vi "ILABW_CaseHandler.vi"(2 "error In":errorcluster, 4 "data":string, 5 "action":string) -> (0 "errorOut":string, 1 "response":string)   [LabVIEW 2012]
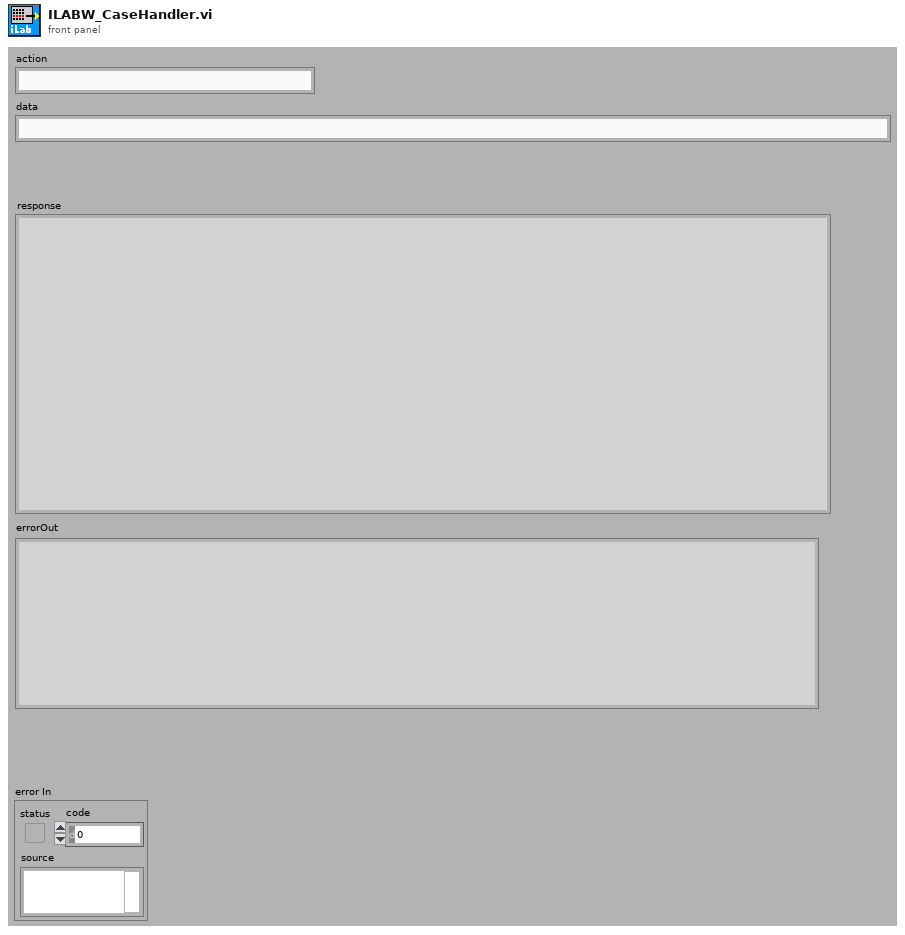
[diagram p1: front panel]
types:
  T1 = enum32{"Bad", "Idle", "Run top level", "Running"}
  T2 = typedef "LVRemotePanelConnectionsTypeDef.ctl" = cluster{"VI Name":string, "Remote":string, "UserName":string, "Port":i32, "Status":enum32{"Viewing", "Waiting For Control", "Controlling"}, "Create Time":timestamp, "Status Time":timestamp, "Control End Time":timestamp}[]
  T3 = cluster{"VI Name":string, "Remote":string, "UserName":string, "Port":i32, "Status":enum32{"Viewing", "Waiting For Control", "Controlling"}, "Create Time":timestamp, "Status Time":timestamp, "Control End Time":timestamp}
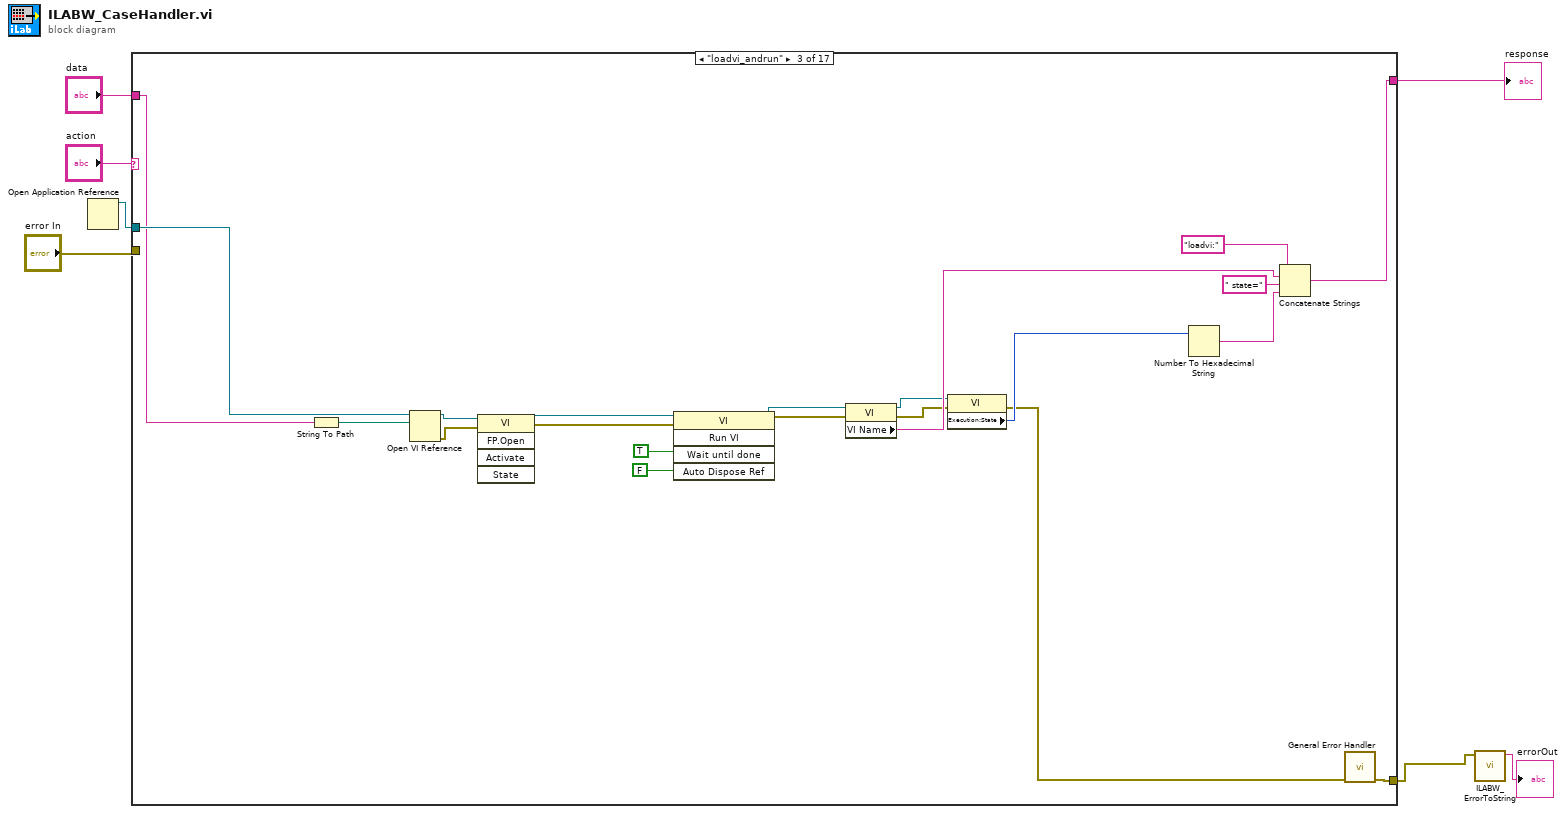
[diagram p0: block diagram]
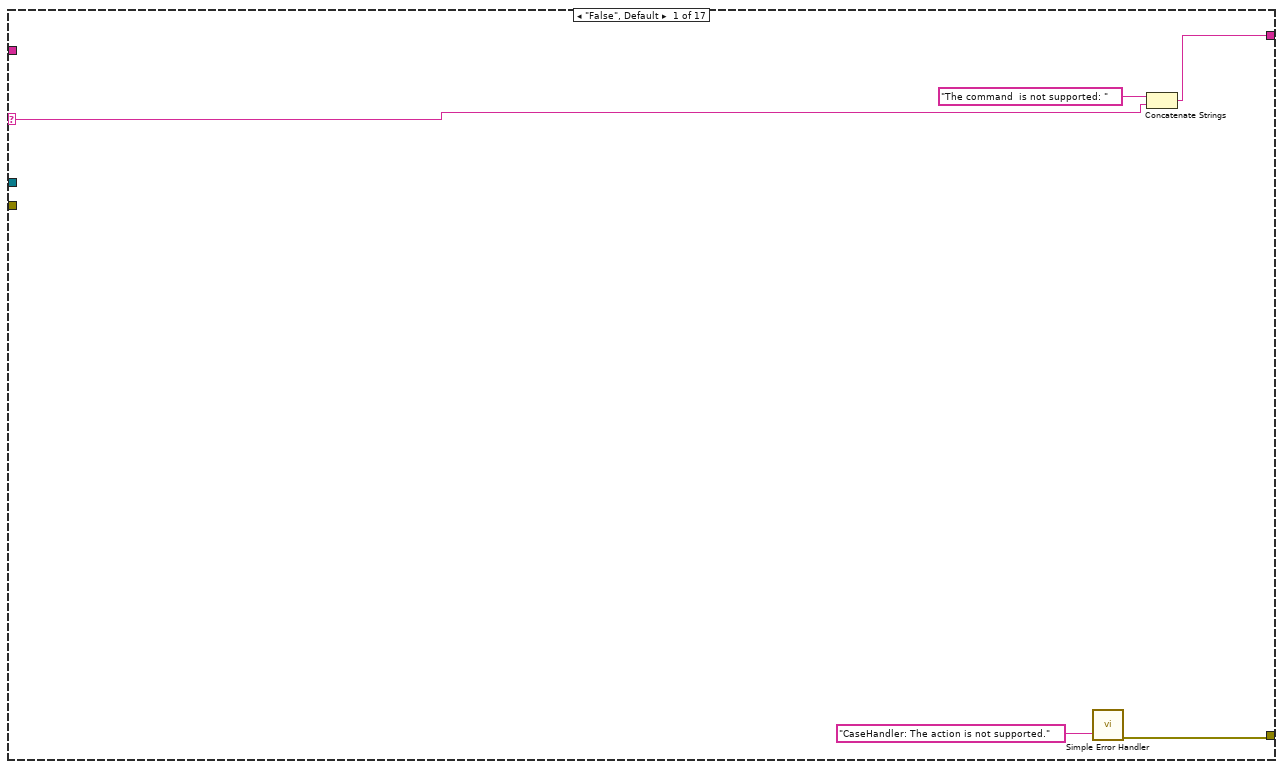
[diagram p2: hidden frame]
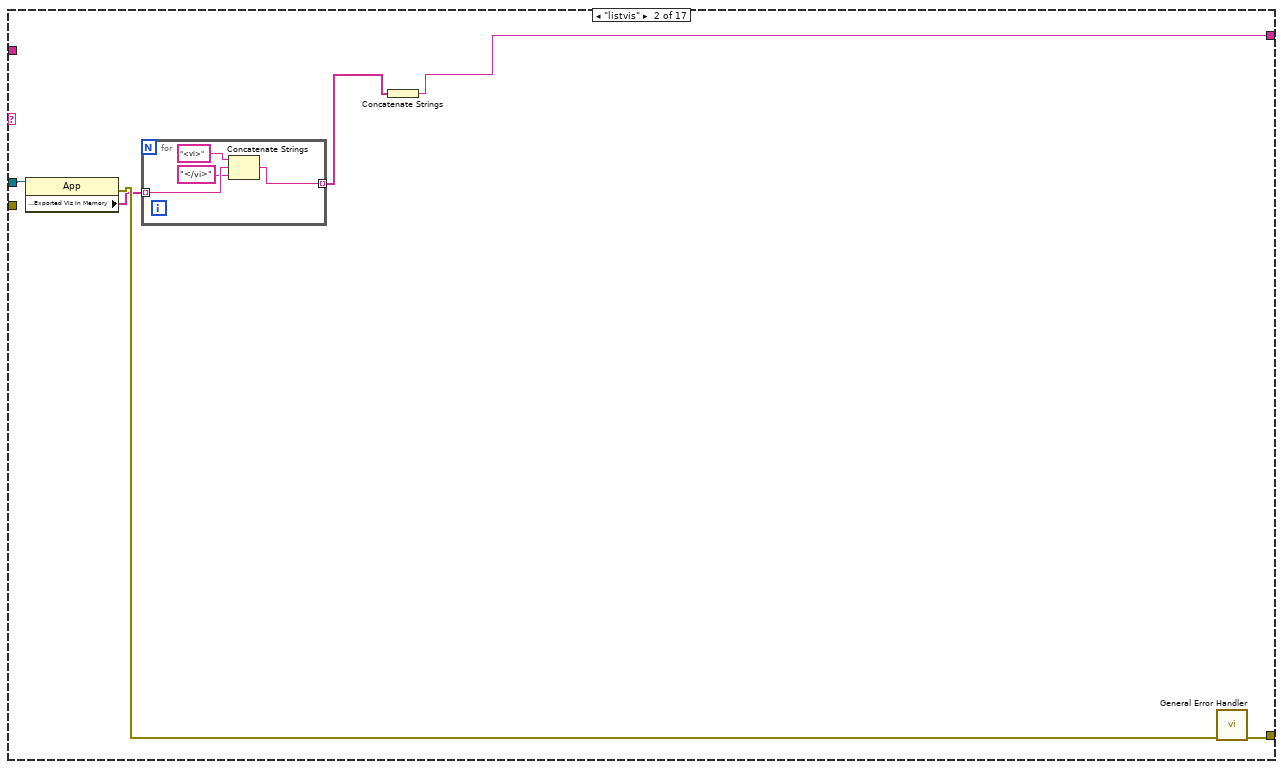
[diagram p3: hidden frame]
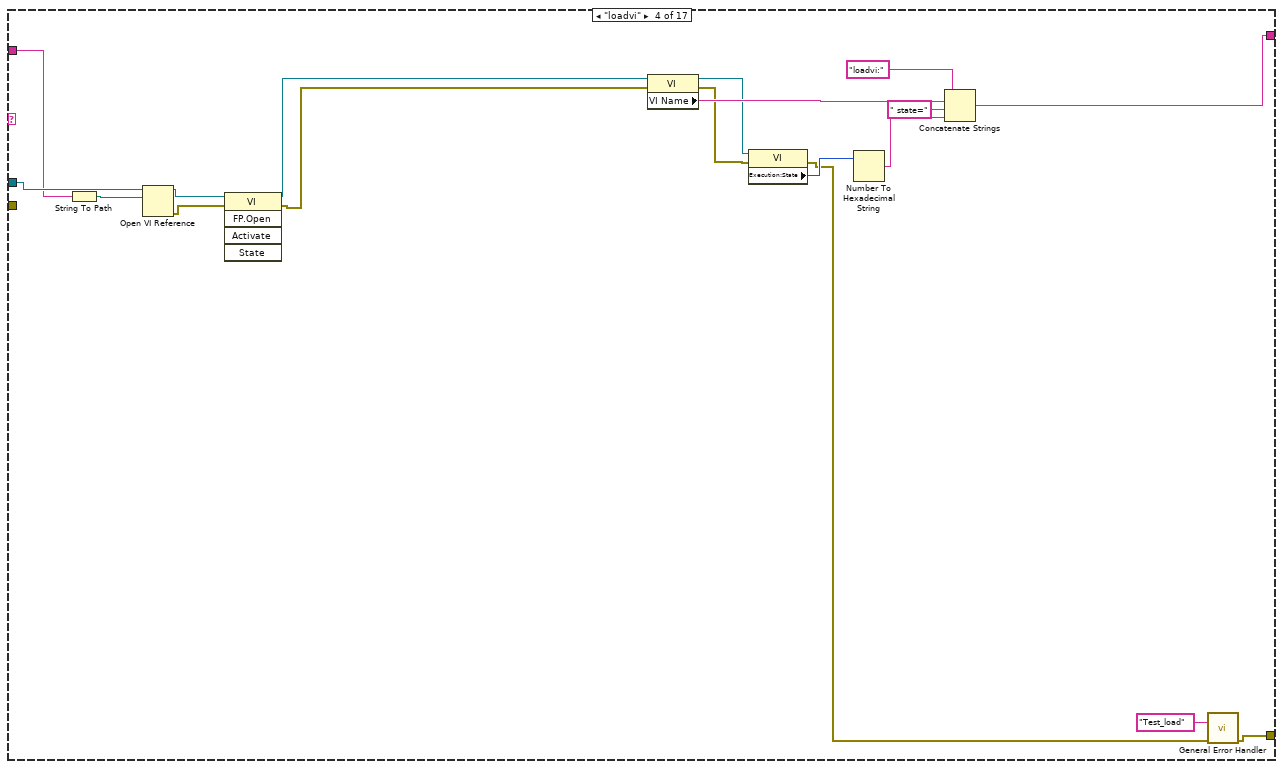
[diagram p4: hidden frame]
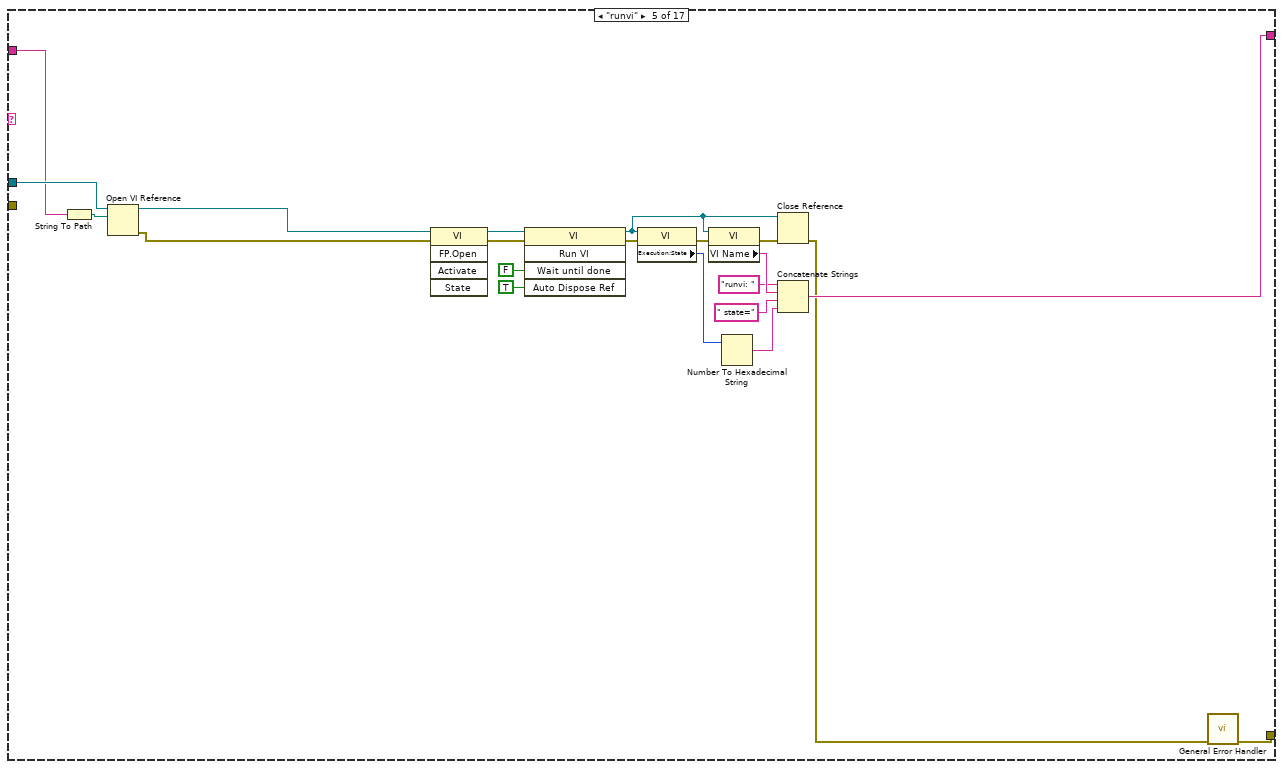
[diagram p5: hidden frame]
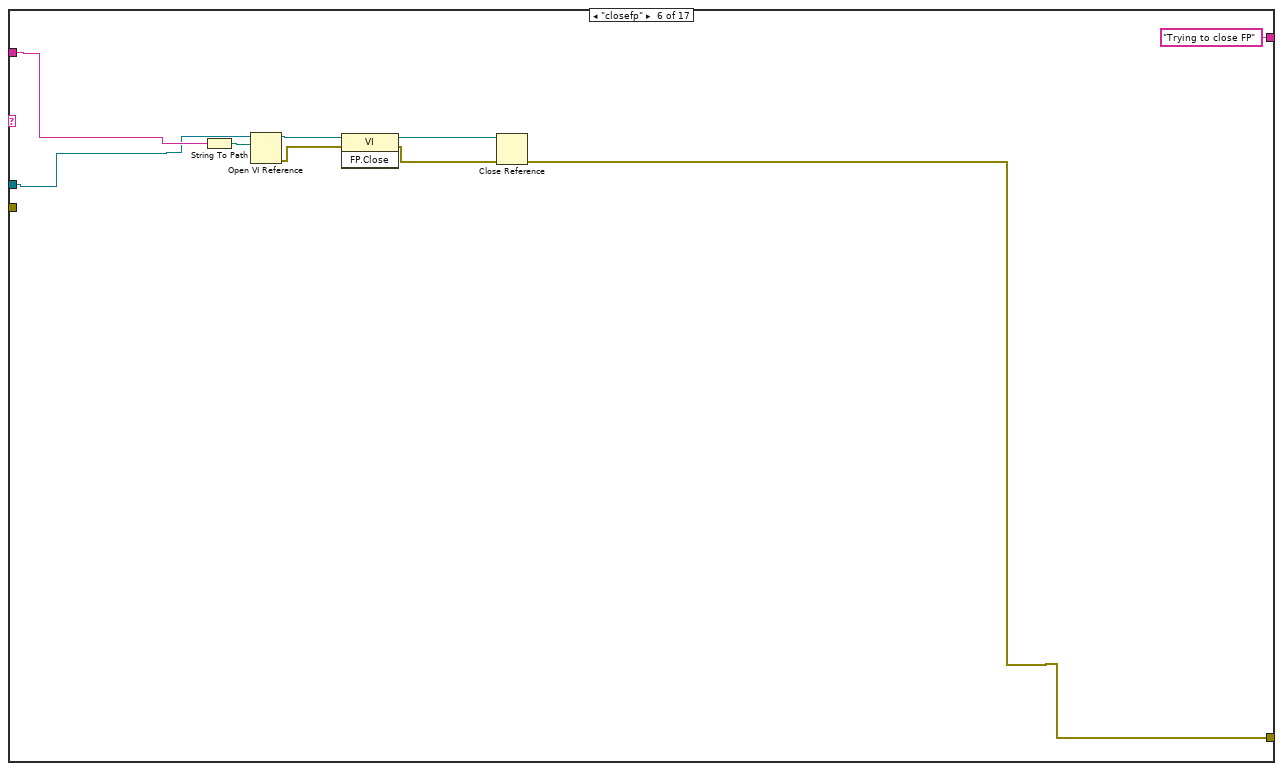
[diagram p6: hidden frame]
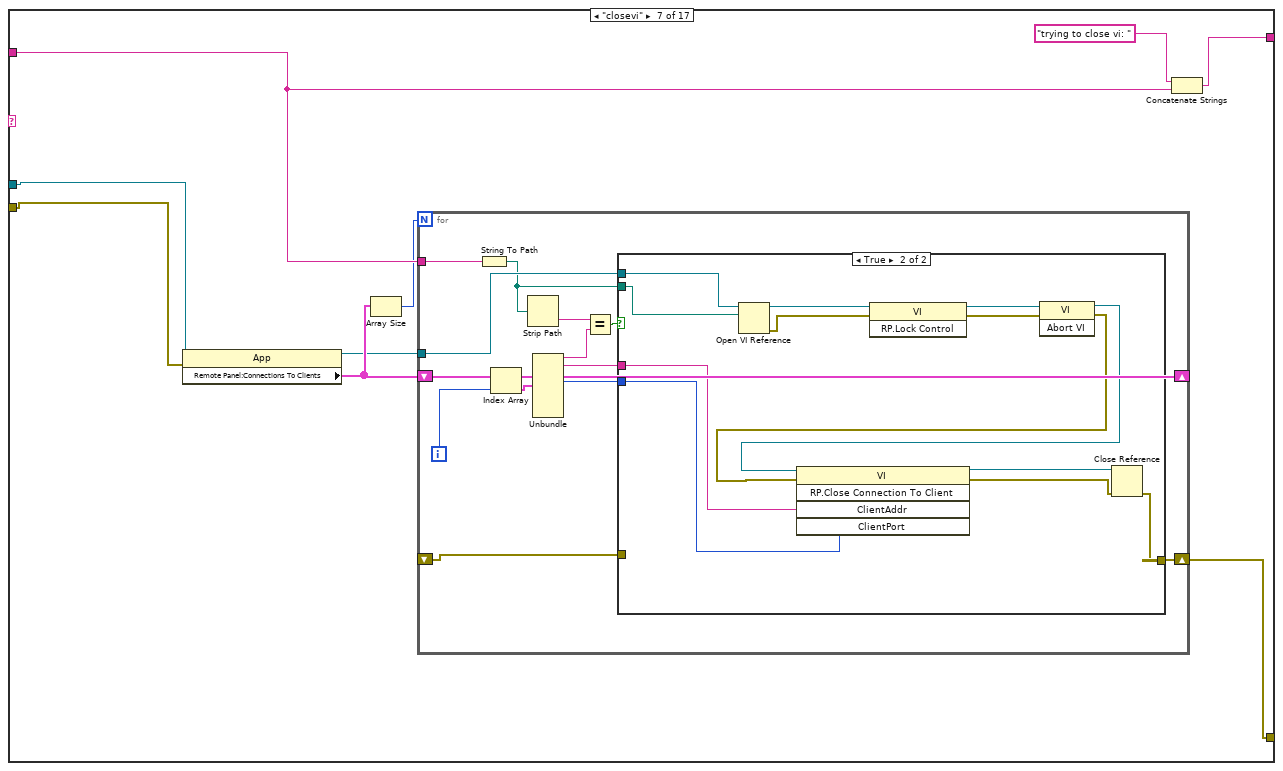
[diagram p7: hidden frame]
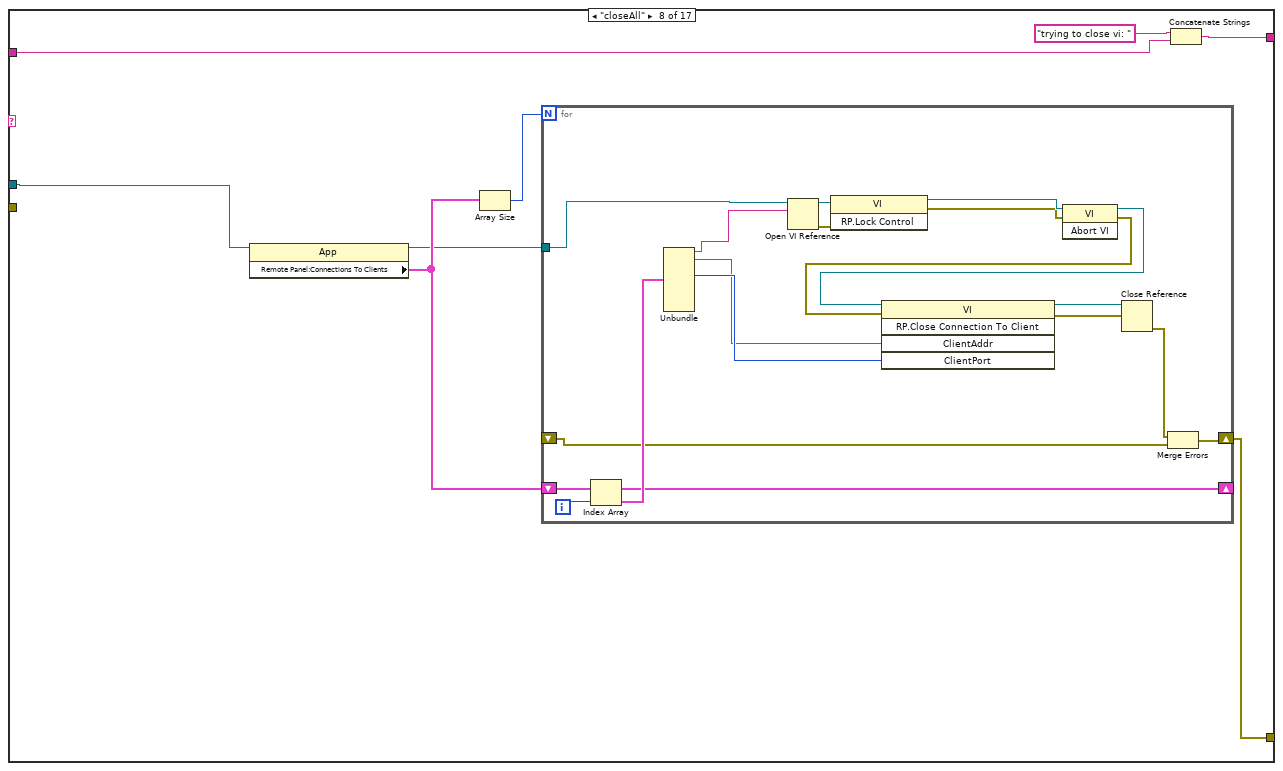
[diagram p9: hidden frame]
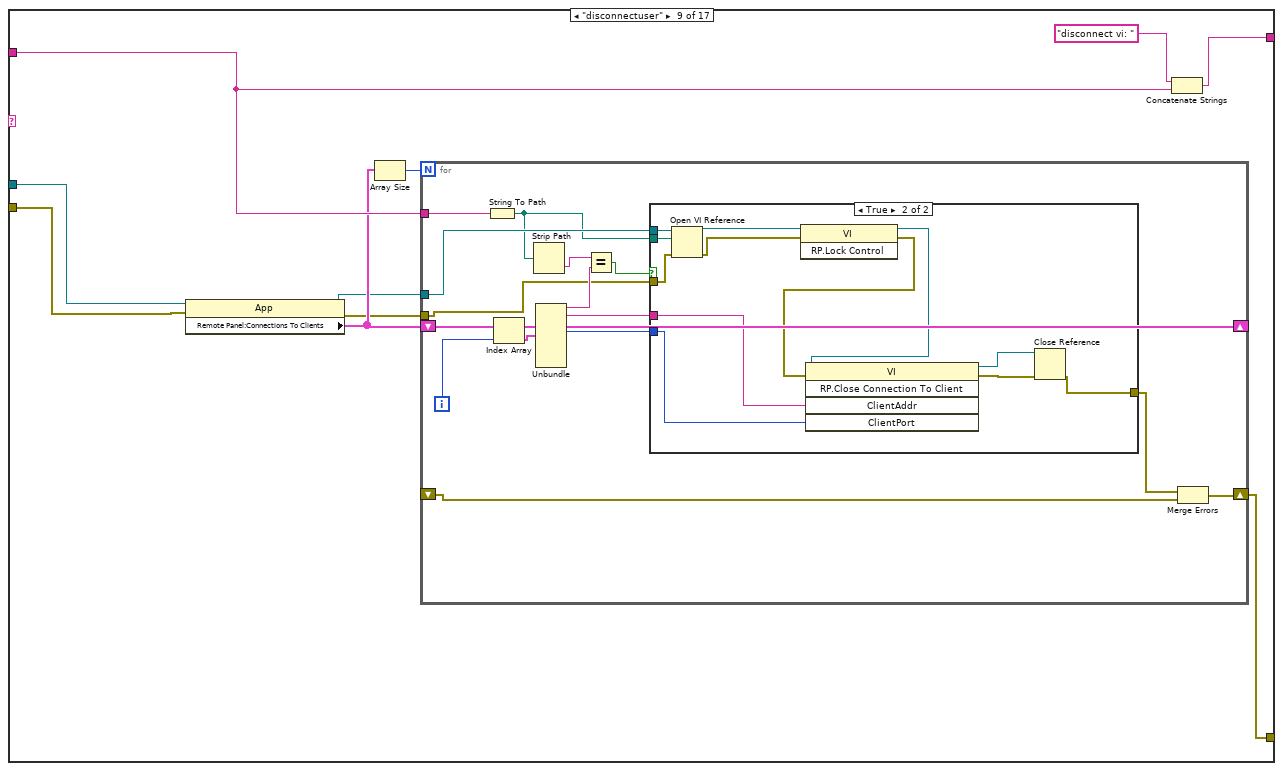
[diagram p10: hidden frame]
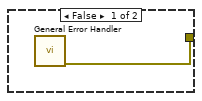
[diagram p11: hidden frame]
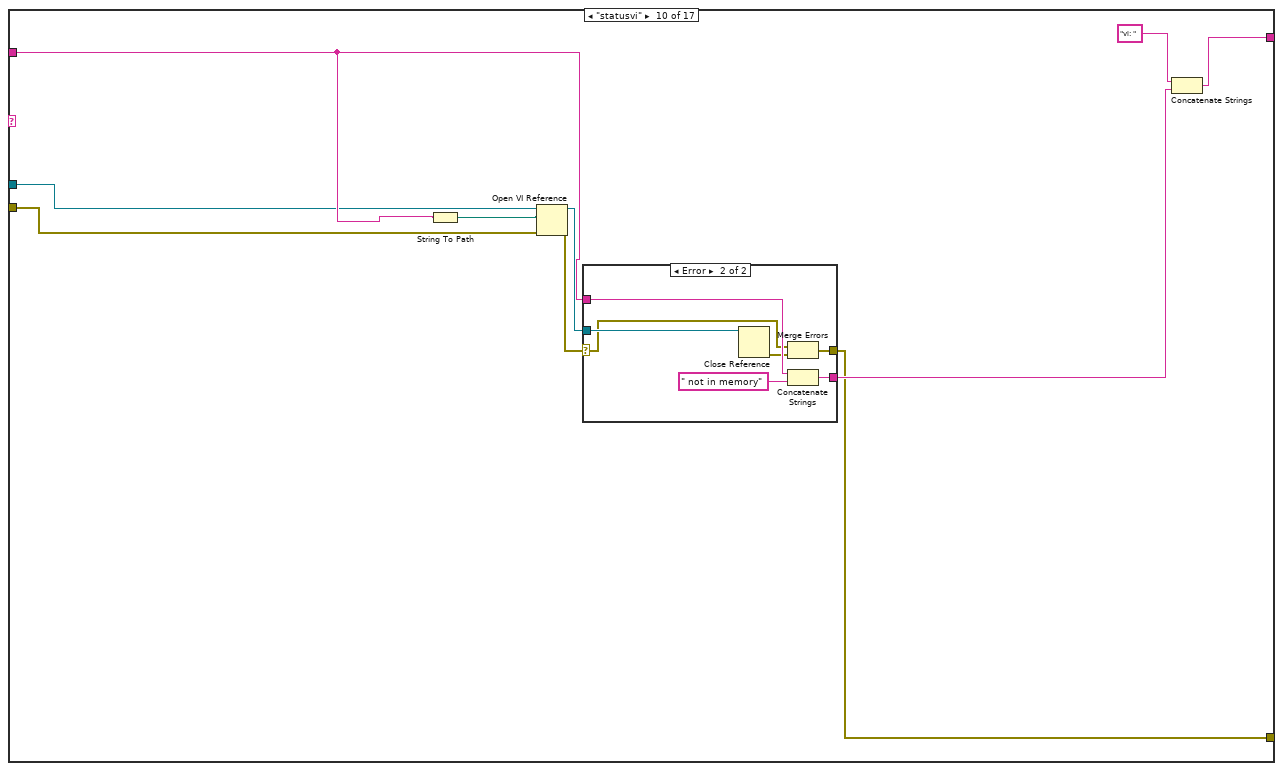
[diagram p12: hidden frame]
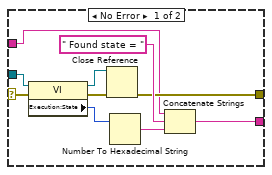
[diagram p13: hidden frame]
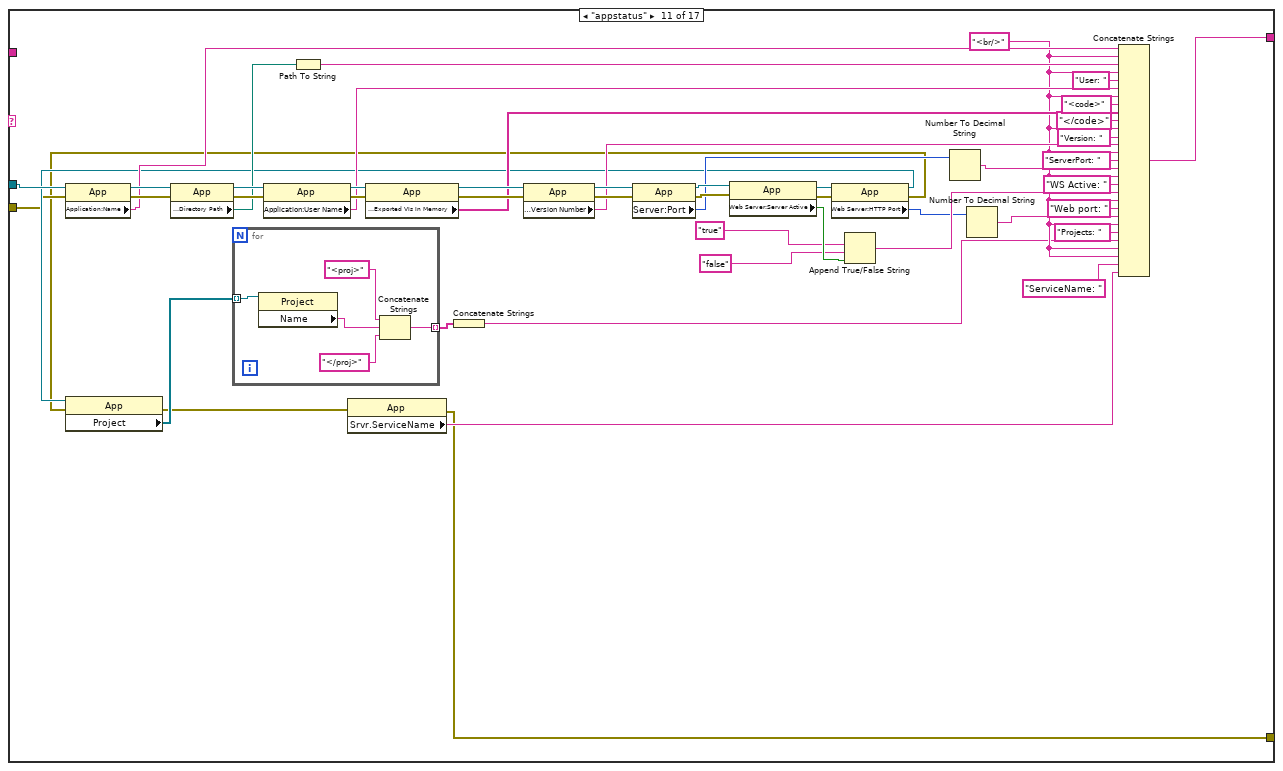
[diagram p14: hidden frame]
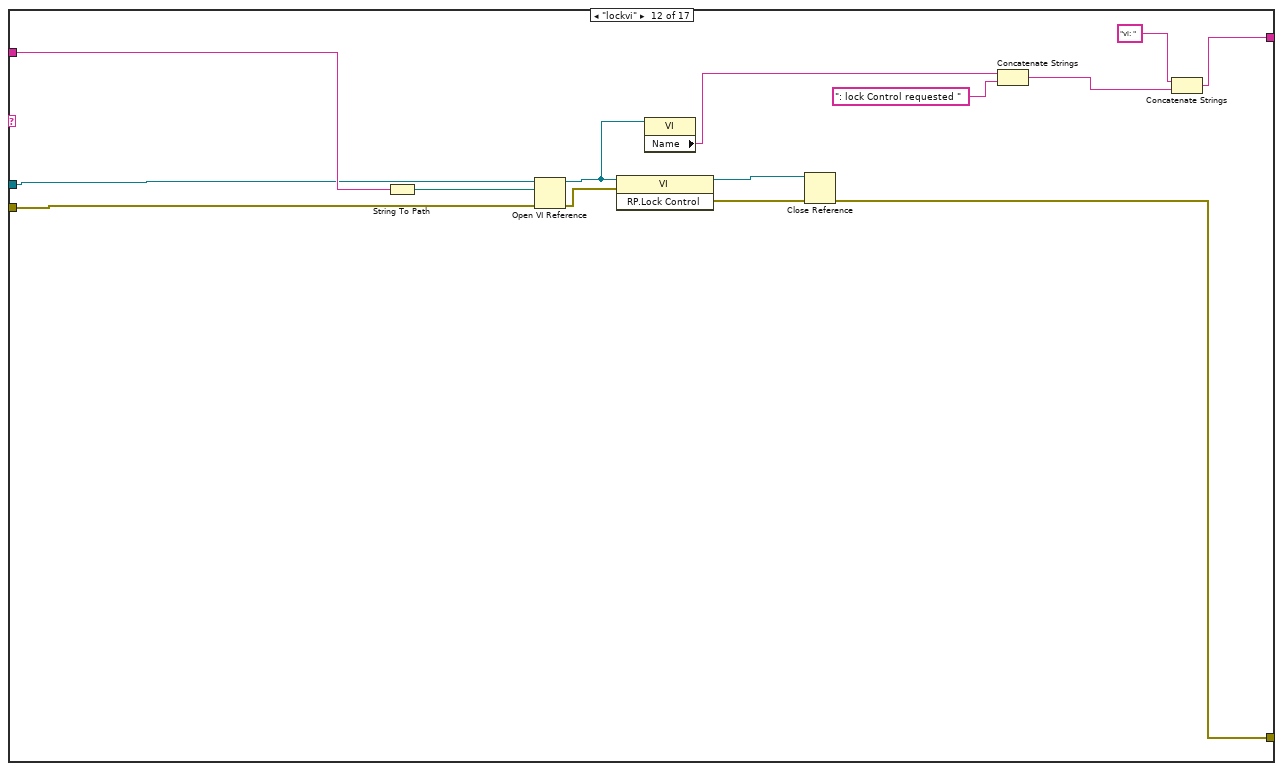
[diagram p15: hidden frame]
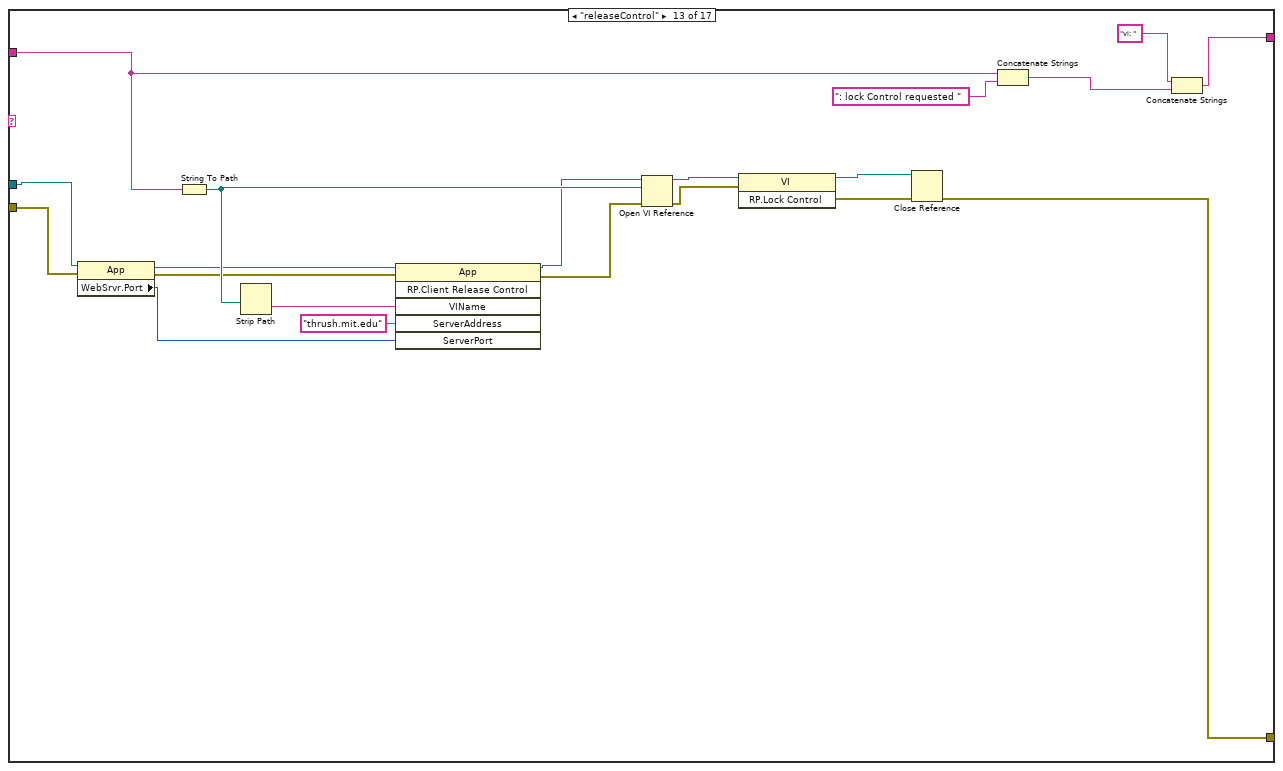
[diagram p16: hidden frame]
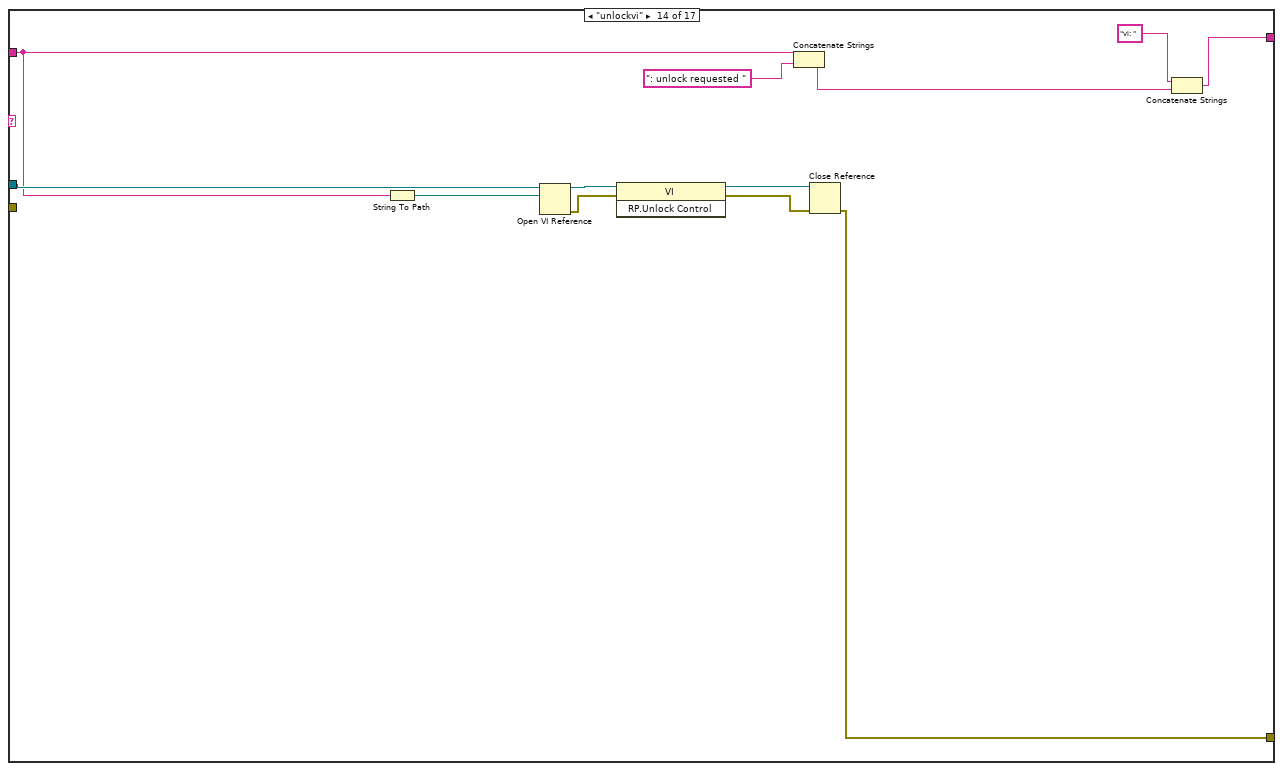
[diagram p17: hidden frame]
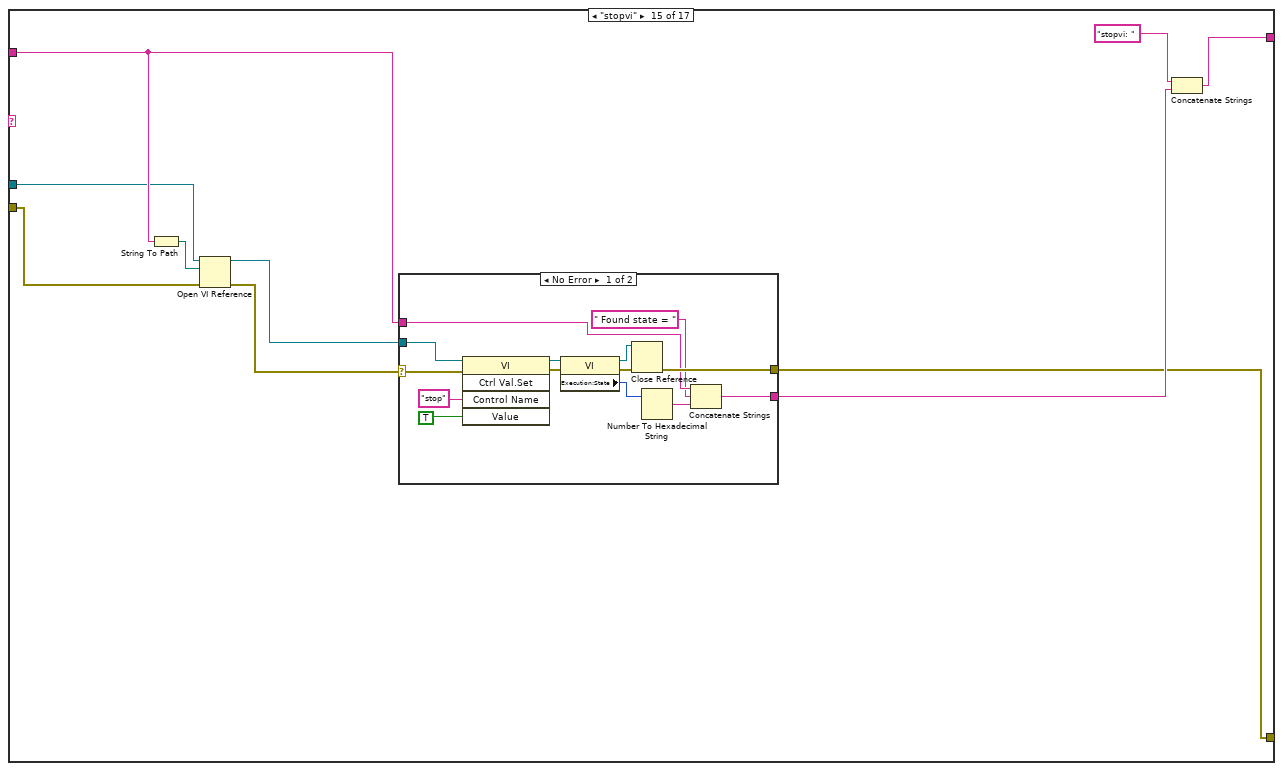
[diagram p18: hidden frame]
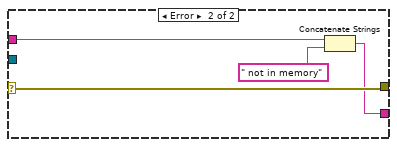
[diagram p19: hidden frame]
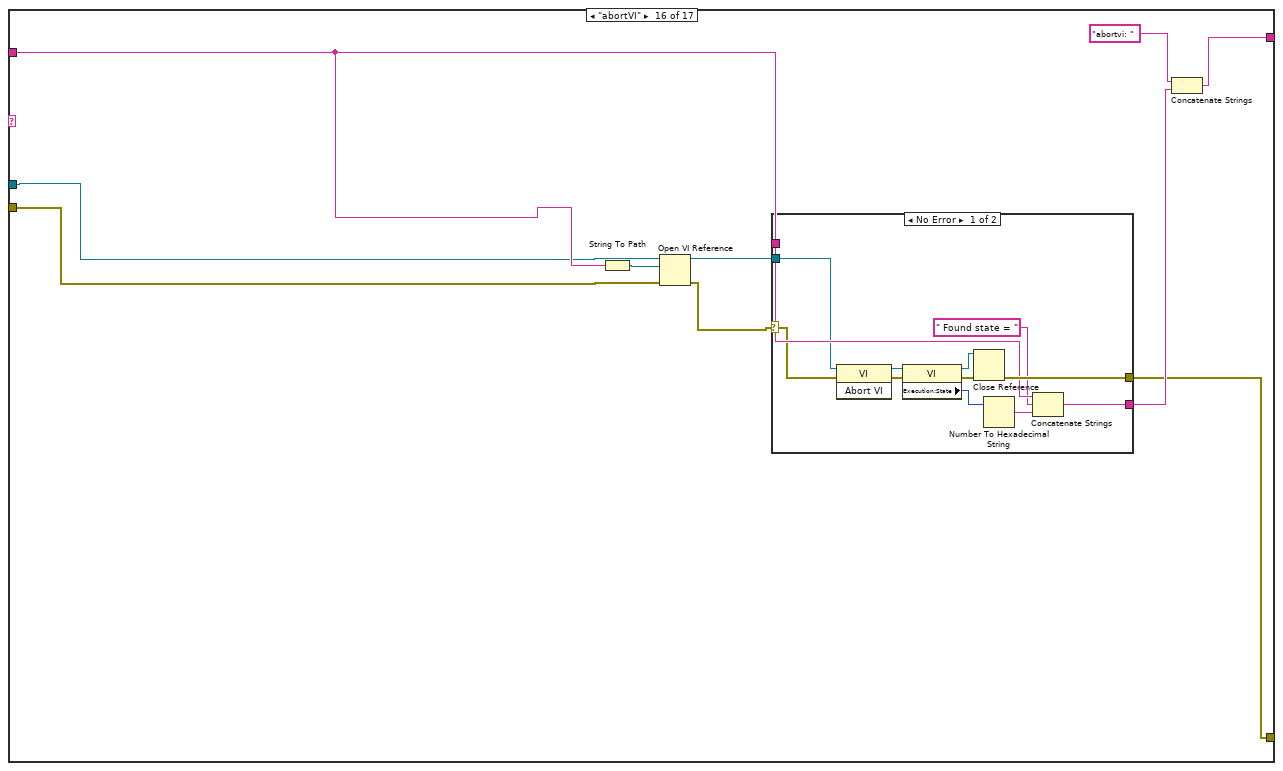
[diagram p20: hidden frame]
diagram:
  n1 = Open Application Reference() -> (3:w5:refnum<vi>)  [unwired: 4 in, 1 out]
  n2 = case shown="\"loadvi_andrun\"" "action" {
    selector: "action" -> [w11 _ _ _ _ _ _ _ _ _ _ _ _ _ _ _ _]
    tunnel: "data" -> [_ _ w24 w44 w66 w91 w97 w132 w160 w198 _ w276 w297 w307 w324 w352 w374]
    tunnel: [w10 w13 w35 w55 w73 "Trying to close FP" ("data") w99 w131 w162 w201 w231 w286 w306 w318 w328 w356 w374] -> w3
    tunnel: [w8 w17 w33 w54 w70 w89 w98 w130 w161 w197 w219 w278 w298 w309 w325 w353 _] -> w1
    tunnel: w5 -> [_ w16 w32 w53 w69 w90 w96 w129 w159 w196 w267 w275 w291 w310 w323 w351 _]
    tunnel: "error In" -> [_ _ _ _ _ _ w95 _ w158 w195 w225 w280 w292 _ w322 w350 _]
    frame "False", Default {
      (unwired) "The" ("message")
      n3 = call <vilib>:"Simple Error Handler.vi"("error source (\" \")"="CaseHandler: The action is not supported." ("error source (\" \")")) -> ("error out"=w8:errorcluster)  [unwired: 2 in, 6 out]
      n4 = Concatenate Strings("The command  is not supported: " ("string"), w11) -> (w10:string)
    }
    frame "listvis" {
      n5 = property class="App"(reference=w16) -> (error out=w18:errorcluster, "Application:Exported VIs In Memory"=w15:string[])  [unwired: 1 in, 1 out]
      n6 = for {
        tunnel: w15 -> [w22] mode=indexing
        tunnel: [w19] -> w14 mode=indexing
        n7 = Concatenate Strings("<vi>" ("string"), w22, "</vi>" ("string")) -> (w19:string)
      }
      n8 = Concatenate Strings(w14) -> (w13:string)
      n9 = call <vilib>:"General Error Handler.vi"("error in (no error)"=w18) -> ("error out"=w17:errorcluster)  [unwired: 1 in, 13 out]
    }
    frame "loadvi_andrun" {
      n10 = String To Path(string=w24) -> (path=w25:path)
      n11 = Open VI Reference(application reference (local)=w32, vi path=w25) -> (vi reference=w42:refnum<vi>, error out=w41:errorcluster)  [unwired: 1 in, 3 out]
      n12 = invoke class="VI" method="FP.Open"(reference=w42, error in=w41) -> (reference out=w31:refnum<vi>, error out=w30:errorcluster)  [unwired: 3 in, 3 out]
      n13 = invoke class="VI" method="Run VI"(reference=w31, error in=w30, "Wait until done"=FALSE, "Auto Dispose Ref"=TRUE) -> (reference out=w29:refnum<vi>, error out=w28:errorcluster)  [unwired: 1 in, 3 out]
      n14 = property class="VI"(reference=w29, error in=w28) -> (reference out=w27:refnum<vi>, error out=w26:errorcluster, "VI Name"=w40:string)
      n15 = property class="VI"(reference=w27, error in=w26) -> (error out=w23:errorcluster, "Execution:State"=w38:T1)  [unwired: 1 out]
      n16 = Number To Hexadecimal String(2:w38) -> (0:w37:string)  [unwired: 1 out]
      n17 = Concatenate Strings("loadvi:" ("string"), w40, " state=" ("string"), w37) -> (w35:string)
      n18 = call <vilib>:"General Error Handler.vi"("error in (no error)"=w23) -> ("error out"=w33:errorcluster)  [unwired: 1 in, 13 out]
    }
    frame "loadvi" {
      n19 = String To Path(string=w44) -> (path=w45:path)
      n20 = Open VI Reference(application reference (local)=w53, vi path=w45) -> (vi reference=w49:refnum<vi>, error out=w48:errorcluster)  [unwired: 1 in, 3 out]
      n21 = invoke class="VI" method="FP.Open"(reference=w49, error in=w48) -> (reference out=w47:refnum<vi>, error out=w46:errorcluster)  [unwired: 3 in, 3 out]
      n22 = property class="VI"(reference=w47, error in=w46) -> (reference out=w51:refnum<vi>, error out=w52:errorcluster, "VI Name"=w60:string)
      n23 = property class="VI"(reference=w51, error in=w52) -> (error out=w50:errorcluster, "Execution:State"=w58:T1)  [unwired: 1 out]
      n24 = Number To Hexadecimal String(2:w58) -> (0:w57:string)  [unwired: 1 out]
      n25 = Concatenate Strings("loadvi:" ("string"), w60, " state=" ("string"), w57) -> (w55:string)
      n26 = call <vilib>:"General Error Handler.vi"("[error source] (\" \")"="Test_load" ("[error source] (\" \")"), "error in (no error)"=w50) -> ("error out"=w54:errorcluster)  [unwired: 1 in, 12 out]
    }
    frame "runvi" {
      w71 = TRUE items=["OFF", "ON", "OFF", "ON"] ("Auto Dispose Ref")
      n27 = String To Path(string=w66) -> (path=w67:path)
      n28 = Open VI Reference(application reference (local)=w69, vi path=w67) -> (vi reference=w81:refnum<vi>, error out=w79:errorcluster)  [unwired: 1 in, 3 out]
      n29 = invoke class="VI" method="FP.Open"(reference=w81, error in=w79) -> (reference out=w78:refnum<vi>, error out=w80:errorcluster)  [unwired: 3 in, 3 out]
      n30 = invoke class="VI" method="Run VI"(reference=w78, error in=w80, "Wait until done"=FALSE, "Auto Dispose Ref"=w71) -> (reference out=w65:refnum<vi>, error out=w64:errorcluster)  [unwired: 1 in, 3 out]
      n31 = property class="VI"(reference=w65, error in=w64) -> (error out=w63:errorcluster, "Execution:State"=w75:T1)  [unwired: 1 out]
      n32 = property class="VI"(reference=w65, error in=w63) -> (error out=w62:errorcluster, "VI Name"=w77:string)  [unwired: 1 out]
      n33 = Number To Hexadecimal String(2:w75) -> (0:w74:string)  [unwired: 1 out]
      n34 = Close Reference(reference=w65, error in (no error)=w62) -> (error out=w68:errorcluster)
      n35 = Concatenate Strings("runvi: " ("string"), w77, " state=" ("string"), w74) -> (w73:string)
      n36 = call <vilib>:"General Error Handler.vi"("error in (no error)"=w68) -> ("error out"=w70:errorcluster)  [unwired: 1 in, 13 out]
    }
    frame "closefp" {
      n37 = String To Path(string=w91) -> (path=w84:path)
      n38 = Open VI Reference(application reference (local)=w90, vi path=w84) -> (vi reference=w87:refnum<vi>, error out=w86:errorcluster)  [unwired: 1 in, 3 out]
      n39 = invoke class="VI" method="FP.Close"(reference=w87, error in=w86) -> (reference out=w83:refnum<vi>, error out=w85:errorcluster)  [unwired: 1 in, 1 out]
      n40 = Close Reference(reference=w83, error in (no error)=w85) -> (error out=w89:errorcluster)
    }
    frame "closevi" {
      n41 = property class="App"(reference=w96, error in=w95) -> (reference out=w92:refnum<vi>, "Remote Panel:Connections To Clients"=w93:T2)  [unwired: 1 out]
      n42 = Array Size(array=w93) -> (size(s)=w94:i32)
      n43 = for {
        N: w94 -> [_]
        shift-right: [w106] -> _
        shift-left: w93 -> [w106]
        tunnel: w97 -> [w103]
        shift-right: [w108] -> w98
        shift-left: _ -> [w101]
        tunnel: w92 -> [w105]
        i -> [w113]
        n44 = String To Path(string=w103) -> (path=w102:path)
        n45 = Index Array(array=w106, index=w113) -> (element=w112:T3)
        n46 = Strip Path(path=w102) -> (name=w104:string)  [unwired: 1 out]
        n47 = Unbundle(w112) -> ("VI Name"=w107:string, "Remote"=w109:string, "Port"=w110:i32)  [unwired: 5 out]
        n48 = Equal?(x=w104, y=w107) -> (x = y?=w111:bool)
        n49 = case shown="True" w111 {
          tunnel: w110 -> [_ w127]
          tunnel: w109 -> [_ w126]
          tunnel: [w114 w125] -> w108
          tunnel: w105 -> [_ w116]
          tunnel: w102 -> [_ w115]
          tunnel: w101 -> [w114 _]
          frame False {
          }
          frame True {
            n50 = Open VI Reference(application reference (local)=w116, vi path=w115) -> (vi reference=w124:refnum<vi>, error out=w123:errorcluster)  [unwired: 1 in, 3 out]
            n51 = invoke class="VI" method="RP.Lock Control"(reference=w124, error in=w123) -> (reference out=w122:refnum<vi>, error out=w121:errorcluster)  [unwired: 1 in, 1 out]
            n52 = invoke class="VI" method="Abort VI"(reference=w122, error in=w121) -> (reference out=w118:refnum<vi>, error out=w120:errorcluster)  [unwired: 1 in, 1 out]
            n53 = invoke class="VI" method="RP.Close Connection To Client"(reference=w118, error in=w120, "ClientAddr"=w126, "ClientPort"=w127) -> (reference out=w117:refnum<vi>, error out=w119:errorcluster)  [unwired: 1 in, 3 out]
            n54 = Close Reference(reference=w117, error in (no error)=w119) -> (error out=w125:errorcluster)
          }
        }
      }
      n55 = Concatenate Strings("trying to close vi: " ("data"), w97) -> (w99:string)
    }
    frame "closeAll" {
      n56 = property class="App"(reference=w129) -> (reference out=w128:refnum<vi>, "Remote Panel:Connections To Clients"=w134:T2)  [unwired: 1 in, 1 out]
      n57 = Array Size(array=w134) -> (size(s)=w135:i32)
      n58 = for {
        N: w135 -> [_]
        shift-right: [w148] -> _
        shift-left: w134 -> [w148]
        shift-right: [w136] -> w130
        shift-left: _ -> [w137]
        tunnel: w128 -> [w147]
        i -> [w153]
        n59 = Index Array(array=w148, index=w153) -> (element=w152:T3)
        n60 = Unbundle(w152) -> ("VI Name"=w149:string, "Remote"=w150:string, "Port"=w151:i32)  [unwired: 5 out]
        n61 = Open VI Reference(application reference (local)=w147, vi path=w149) -> (vi reference=w142:refnum<vi>, error out=w141:errorcluster)  [unwired: 1 in, 3 out]
        n62 = invoke class="VI" method="RP.Lock Control"(reference=w142, error in=w141) -> (reference out=w140:refnum<vi>, error out=w139:errorcluster)  [unwired: 1 in, 1 out]
        n63 = invoke class="VI" method="Abort VI"(reference=w140, error in=w139) -> (reference out=w143:refnum<vi>, error out=w144:errorcluster)  [unwired: 1 in, 1 out]
        n64 = invoke class="VI" method="RP.Close Connection To Client"(reference=w143, error in=w144, "ClientAddr"=w150, "ClientPort"=w151) -> (reference out=w146:refnum<vi>, error out=w145:errorcluster)  [unwired: 1 in, 3 out]
        n65 = Close Reference(reference=w146, error in (no error)=w145) -> (error out=w138:errorcluster)
        n66 = Merge Errors(w138, w137) -> (w136:errorcluster)
      }
      n67 = Concatenate Strings("trying to close vi: " ("data"), w132) -> (w131:string)
    }
    frame "disconnectuser" {
      n68 = property class="App"(reference=w159, error in=w158) -> (reference out=w155:refnum<vi>, error out=w154:errorcluster, "Remote Panel:Connections To Clients"=w156:T2)
      n69 = Array Size(array=w156) -> (size(s)=w157:i32)
      n70 = for {
        N: w157 -> [_]
        shift-right: [w172] -> _
        shift-left: w156 -> [w172]
        tunnel: w160 -> [w168]
        shift-right: [w165] -> w161
        shift-left: _ -> [w164]
        tunnel: w155 -> [w171]
        tunnel: w154 -> [w170]
        i -> [w178]
        n71 = String To Path(string=w168) -> (path=w167:path)
        n72 = Index Array(array=w172, index=w178) -> (element=w177:T3)
        n73 = Strip Path(path=w167) -> (name=w169:string)  [unwired: 1 out]
        n74 = Unbundle(w177) -> ("VI Name"=w173:string, "Remote"=w174:string, "Port"=w175:i32)  [unwired: 5 out]
        n75 = Equal?(x=w169, y=w173) -> (x = y?=w176:bool)
        n76 = case shown="True" w176 {
          tunnel: w175 -> [_ w191]
          tunnel: w174 -> [_ w190]
          tunnel: [w179 w182] -> w166
          tunnel: w171 -> [_ w185]
          tunnel: w170 -> [_ w181]
          tunnel: w167 -> [_ w180]
          frame False {
            n77 = call <vilib>:"General Error Handler.vi"() -> ("error out"=w179:errorcluster)  [unwired: 2 in, 13 out]
          }
          frame True {
            n78 = Open VI Reference(application reference (local)=w185, vi path=w180, error in (no error)=w181) -> (vi reference=w189:refnum<vi>, error out=w186:errorcluster)  [unwired: 3 out]
            n79 = invoke class="VI" method="RP.Lock Control"(reference=w189, error in=w186) -> (reference out=w188:refnum<vi>, error out=w187:errorcluster)  [unwired: 1 in, 1 out]
            n80 = invoke class="VI" method="RP.Close Connection To Client"(reference=w188, error in=w187, "ClientAddr"=w190, "ClientPort"=w191) -> (reference out=w183:refnum<vi>, error out=w184:errorcluster)  [unwired: 1 in, 3 out]
            n81 = Close Reference(reference=w183, error in (no error)=w184) -> (error out=w182:errorcluster)
          }
        }
        n82 = Merge Errors(w166, w164) -> (w165:errorcluster)
      }
      n83 = Concatenate Strings("disconnect vi: " ("data"), w160) -> (w162:string)
    }
    frame "statusvi" {
      n84 = String To Path(string=w198) -> (path=w194:path)
      n85 = Open VI Reference(application reference (local)=w196, vi path=w194, error in (no error)=w195) -> (vi reference=w192:refnum<vi>, error out=w193:errorcluster)  [unwired: 3 out]
      n86 = case shown="Error" w193 {
        selector: w193 -> [w202 w213]
        tunnel: w198 -> [w204 w217]
        tunnel: [w206 w212] -> w197
        tunnel: w192 -> [w205 w215]
        tunnel: [w203 w216] -> w199
        frame No Error {
          n87 = property class="VI"(reference=w205, error in=w202) -> (reference out=w210:refnum<vi>, error out=w211:errorcluster, "Execution:State"=w207:T1)
          n88 = Close Reference(reference=w210, error in (no error)=w211) -> (error out=w206:errorcluster)
          n89 = Number To Hexadecimal String(2:w207) -> (0:w208:string)  [unwired: 1 out]
          n90 = Concatenate Strings(w204, " Found state = " ("string"), w208) -> (w203:string)
        }
        frame Error {
          n91 = Close Reference(reference=w215) -> (error out=w214:errorcluster)  [unwired: 1 in]
          n92 = Merge Errors(w213, w214) -> (w212:errorcluster)
          n93 = Concatenate Strings(w217, " not in memory" ("string")) -> (w216:string)
        }
      }
      n94 = Concatenate Strings("vi: " ("data"), w199) -> (w201:string)
    }
    frame "appstatus" {
      w228 = "<br/>" ("string")
      n95 = property class="App"(reference=w267, error in=w225) -> (reference out=w266:refnum<vi>, error out=w261:errorcluster, "Application:Name"=w252:string)
      n96 = property class="App"(reference=w266, error in=w261) -> (reference out=w265:refnum<vi>, error out=w260:errorcluster, "Application:Directory Path"=w250:path)
      n97 = property class="App"(reference=w265, error in=w260) -> (reference out=w264:refnum<vi>, error out=w259:errorcluster, "Application:User Name"=w248:string)
      n98 = Path To String(path=w250) -> (string=w251:string)
      n99 = property class="App"(reference=w264, error in=w259) -> (reference out=w263:refnum<vi>, error out=w258:errorcluster, "Application:Exported VIs In Memory"=w246:string[])
      n100 = property class="App"(reference=w263, error in=w258) -> (reference out=w262:refnum<vi>, error out=w257:errorcluster, "Application:Version Number"=w243:string)
      n101 = property class="App"(reference=w262, error in=w257) -> (reference out=w253:refnum<vi>, error out=w254:errorcluster, "Server:Port"=w240:u32)
      n102 = property class="App"(reference=w253, error in=w254) -> (reference out=w256:refnum<vi>, error out=w255:errorcluster, "Web Server:Server Active"=w238:bool)
      n103 = property class="App"(reference=w256, error in=w255) -> (reference out=w230:refnum<vi>, error out=w221:errorcluster, "Web Server:HTTP Port"=w233:u16)
      n104 = property class="App"(reference=w230, error in=w221) -> (error out=w220:errorcluster, "Project"=w224:refnum<vi>[])  [unwired: 1 out]
      n105 = for {
        tunnel: w224 -> [w272] mode=indexing
        tunnel: [w268] -> w223 mode=indexing
        n106 = property class="Project"(reference=w272) -> ("Name"=w271:string)  [unwired: 1 in, 2 out]
        n107 = Concatenate Strings("<proj>" ("string"), w271, "</proj>" ("string")) -> (w268:string)
      }
      n108 = property class="App"(error in=w220) -> (error out=w219:errorcluster, "Srvr.ServiceName"=w226:string)  [unwired: 1 in, 1 out]
      n109 = Concatenate Strings(w223) -> (w222:string)
      n110 = Append True/False String(1:w238, 2:"false" ("false string"), 3:"true" ("true string")) -> (0:w237:string)  [unwired: 1 out]
      n111 = Number To Decimal String(number=w240) -> (decimal integer string=w241:string)  [unwired: 1 out]
      n112 = Number To Decimal String(number=w233) -> (decimal integer string=w232:string)  [unwired: 1 out]
      n113 = Concatenate Strings(w252, w228, w251, w228, "User: " ("string"), w248, w228, "<code>" ("string"), w246, "</code>" ("string"), w228, "Version: " ("string"), w243, w228, "ServerPort: " ("string"), w241, w228, "WS Active: " ("string"), w237, w228, "Web port: " ("string"), w232, w228, "Projects: " ("string"), w222, w228, w228, "ServiceName: " ("string"), w226) -> (w231:string)
    }
    frame "lockvi" {
      n114 = String To Path(string=w276) -> (path=w277:path)
      n115 = Open VI Reference(application reference (local)=w275, vi path=w277, error in (no error)=w280) -> (vi reference=w274:refnum<vi>, error out=w284:errorcluster)  [unwired: 3 out]
      n116 = invoke class="VI" method="RP.Lock Control"(reference=w274, error in=w284) -> (reference out=w282:refnum<vi>, error out=w281:errorcluster)  [unwired: 1 in, 1 out]
      n117 = property class="VI"(reference=w274) -> ("Name"=w273:string)  [unwired: 1 in, 2 out]
      n118 = Close Reference(reference=w282, error in (no error)=w281) -> (error out=w278:errorcluster)
      n119 = Concatenate Strings(w273, ": lock Control requested " ("string")) -> (w279:string)
      n120 = Concatenate Strings("vi: " ("data"), w279) -> (w286:string)
    }
    frame "releaseControl" {
      n121 = property class="App"(reference=w291, error in=w292) -> (reference out=w290:refnum<vi>, error out=w287:errorcluster, "WebSrvr.Port"=w294:u16)
      n122 = String To Path(string=w297) -> (path=w296:path)
      n123 = Strip Path(path=w296) -> (name=w295:string)  [unwired: 1 out]
      n124 = invoke class="App" method="RP.Client Release Control"(reference=w290, error in=w287, "VIName"=w295, "ServerAddress"="thrush.mit.edu" ("Server Address"), "ServerPort"=w294) -> (reference out=w288:refnum<vi>, error out=w289:errorcluster)  [unwired: 1 in, 4 out]
      n125 = Open VI Reference(application reference (local)=w288, vi path=w296, error in (no error)=w289) -> (vi reference=w304:refnum<vi>, error out=w303:errorcluster)  [unwired: 3 out]
      n126 = invoke class="VI" method="RP.Lock Control"(reference=w304, error in=w303) -> (reference out=w301:refnum<vi>, error out=w300:errorcluster)  [unwired: 1 in, 1 out]
      n127 = Close Reference(reference=w301, error in (no error)=w300) -> (error out=w298:errorcluster)
      n128 = Concatenate Strings(w297, ": lock Control requested " ("string")) -> (w299:string)
      n129 = Concatenate Strings("vi: " ("data"), w299) -> (w306:string)
    }
    frame "unlockvi" {
      n130 = String To Path(string=w307) -> (path=w308:path)
      n131 = Open VI Reference(application reference (local)=w310, vi path=w308) -> (vi reference=w316:refnum<vi>, error out=w315:errorcluster)  [unwired: 1 in, 3 out]
      n132 = invoke class="VI" method="RP.Unlock Control"(reference=w316, error in=w315) -> (reference out=w313:refnum<vi>, error out=w312:errorcluster)  [unwired: 1 in, 1 out]
      n133 = Concatenate Strings(w307, ": unlock requested " ("string")) -> (w311:string)
      n134 = Close Reference(reference=w313, error in (no error)=w312) -> (error out=w309:errorcluster)
      n135 = Concatenate Strings("vi: " ("data"), w311) -> (w318:string)
    }
    frame "stopvi" {
      n136 = String To Path(string=w324) -> (path=w321:path)
      n137 = Open VI Reference(application reference (local)=w323, vi path=w321, error in (no error)=w322) -> (vi reference=w320:refnum<vi>, error out=w319:errorcluster)  [unwired: 1 in, 2 out]
      n138 = case shown="No Error" w319 {
        selector: w319 -> [w329 w346]
        tunnel: [w342 w343] -> w326
        tunnel: [w341 w346] -> w325
        tunnel: w324 -> [w340 w344]
        tunnel: w320 -> [w334 _]
        frame No Error {
          n139 = invoke class="VI" method="Ctrl Val.Set"(reference=w334, error in=w329, "Control Name"="stop", "Value"=TRUE) -> (reference out=w331:refnum<vi>, error out=w332:errorcluster)  [unwired: 1 in, 3 out]
          n140 = property class="VI"(reference=w331, error in=w332) -> (reference out=w336:refnum<vi>, error out=w335:errorcluster, "Execution:State"=w339:T1)
          n141 = Close Reference(reference=w336, error in (no error)=w335) -> (error out=w341:errorcluster)
          n142 = Number To Hexadecimal String(2:w339) -> (0:w338:string)  [unwired: 1 out]
          n143 = Concatenate Strings(w340, " Found state = " ("string"), w338) -> (w342:string)
        }
        frame Error {
          n144 = Concatenate Strings(w344, " not in memory" ("string")) -> (w343:string)
        }
      }
      n145 = Concatenate Strings("stopvi: " ("data"), w326) -> (w328:string)
    }
    frame "abortVI" {
      n146 = String To Path(string=w352) -> (path=w348:path)
      n147 = Open VI Reference(application reference (local)=w351, vi path=w348, error in (no error)=w350) -> (vi reference=w349:refnum<vi>, error out=w347:errorcluster)  [unwired: 1 in, 2 out]
      n148 = case shown="No Error" w347 {
        selector: w347 -> [w357 w372]
        tunnel: [w368 w371] -> w354
        tunnel: [w367 w372] -> w353
        tunnel: w352 -> [w366 w369]
        tunnel: w349 -> [w358 _]
        frame No Error {
          n149 = invoke class="VI" method="Abort VI"(reference=w358, error in=w357) -> (reference out=w362:refnum<vi>, error out=w361:errorcluster)  [unwired: 1 in, 1 out]
          n150 = property class="VI"(reference=w362, error in=w361) -> (reference out=w360:refnum<vi>, error out=w359:errorcluster, "Execution:State"=w365:T1)
          n151 = Close Reference(reference=w360, error in (no error)=w359) -> (error out=w367:errorcluster)
          n152 = Number To Hexadecimal String(2:w365) -> (0:w364:string)  [unwired: 1 out]
          n153 = Concatenate Strings(w366, " Found state = " ("string"), w364) -> (w368:string)
        }
        frame Error {
          n154 = Concatenate Strings(w369, " not in memory" ("string")) -> (w371:string)
        }
      }
      n155 = Concatenate Strings("abortvi: " ("data"), w354) -> (w356:string)
    }
    frame "exit" {
      n156 = Quit LabVIEW(quit? (T)=TRUE) -> ()
    }
  }
  "response" <- w3
  n157 = call "ILABW_ErrorToString.vi"("errorIn"=w1) -> ("errorOut"=→"errorOut":string)  [unwired: 10 in]
